vi "mqttCmdAcknowledge.vi"(0 "_mqtt in":refnum<class "mqttCmdPing.lvclass">, 7 "mqtt in":refnum<class "mqtt.lvclass">, 11 "error in (no error)":errorcluster) -> (4 "_mqtt out":refnum<class "mqttCmdPing.lvclass">, 8 "notification":T1, 15 "error out":errorcluster)   [LabVIEW 2018, in "labview-mqtt.lvlib" / "mqttCmdPing.lvclass"]
uses:
  mqttCmdPing.lvclass
  D:/OneDrive/_WorkingOn/IECube/MQTT LabVIEW/mqtt-LabVIEW-master-yao/src/class/mqtt/mqttCmd/mqttCmd.lvclass
  mqttTypedef/mqttRXdataCluster.ctl
  mqttTypedef/mqttFixedHeaderResponse.ctl
  mqttTypedef/mqttQOSlevel.ctl
  mqttTypedef/mqttMessageType.ctl
  mqtt.lvclass
  mqttCmd.lvclass/mqttCmd.ctl
  labview-mqtt.lvlib
  mqttCmd.lvclass
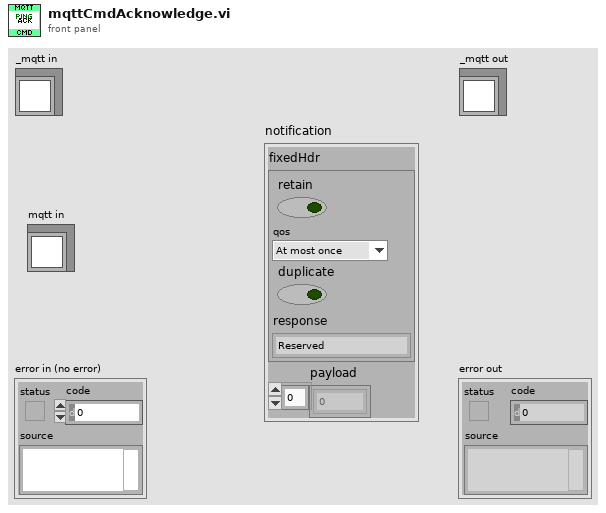
[diagram p1: front panel]
types:
  T1 = typedef "labview-mqtt.lvlib/mqttRXdataCluster.ctl" = cluster{"fixedHdr":T2, "payload":u8[]}
  T2 = typedef "labview-mqtt.lvlib/mqttFixedHeaderResponse.ctl" = cluster{"retain":bool, "qos":T3, "duplicate":bool, "response":T4}
  T3 = typedef "labview-mqtt.lvlib/mqttQOSlevel.ctl" = enum8{"At most once", "At least once", "Exactly once", "Reserved"}
  T4 = typedef "labview-mqtt.lvlib/mqttMessageType.ctl" = enum32{"Reserved", "CONNECT", "CONNACK", "PUBLISH", "PUBACK", "PUBREC", "PUBREL", "PUBCOMP", "SUBSCRIBE", "SUBACK", "UNSUBSCRIBE", "UNSUBACK", "PINGREQ", "PINGRESP", "DISCONNECT", "Reserved2"}
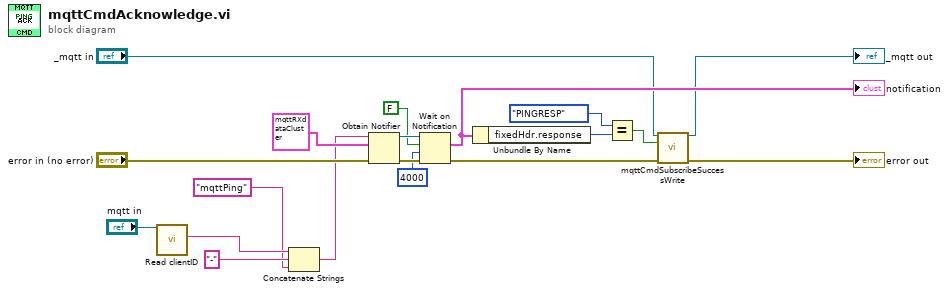
[diagram p0: block diagram]
diagram:
  n1 = call-dynamic "Read clientID.vi"("mqtt in"="mqtt in") -> ("clientID"=w4:string)  [unwired: 8 in, 2 out]
  n2 = Concatenate Strings(w4, "-" ("string"), "mqttPing" ("name (unnamed)")) -> (w1:string)
  n3 = Obtain Notifier(name (unnamed)=w1, notification data type=T1 {"fixedHdr"={"retain"=FALSE, "qos"=enum."At most once", "duplicate"=FALSE, "response"=enum."Reserved"}, "payload"=[]} ("notification"), error in (no error)="error in (no error)") -> (notifier out=w17:refnum<notifier>, error out=w19:errorcluster)  [unwired: 1 in, 1 out]
  n4 = Wait on Notification(notifier=w17, ignore previous (F)=FALSE, timeout in ms (-1)=4000, error in (no error)=w19) -> (notification=w13:T1, error out=w9:errorcluster)  [unwired: 2 out]
  "notification" <- w13
  n5 = Unbundle By Name(w13) -> ("fixedHdr.response"=w12:T4)
  n6 = Equal?(x=mqttMessageType."PINGRESP", y=w12) -> (x = y?=w10:bool)
  n7 = call "mqttCmdSubscribeSuccessWrite.vi"("mqttBrokerCommand in"="_mqtt in", "success"=w10, "error in (no error)"=w9) -> ("mqttBrokerCommand out"=→"_mqtt out":refnum<class "mqttCmdPing.lvclass">, "error out"=→"error out":errorcluster)  [unwired: 11 in]
